vi "Read Channel suffix.vi"(8 "error in (no error)":errorcluster, 11 "Tag Channel Column in":refnum<class "Tag Channel Column.lvclass">) -> (0 "error out":errorcluster, 2 "Channel suffix":string, 3 "Tag Channel Column out":refnum<class "Tag Channel Column.lvclass">)   [LabVIEW 2013, in "Table Manager.lvlib" / "Tag Channel Column.lvclass"]
uses:
  Tag Channel Column.lvclass
  Tag Channel Column.lvclass/Tag Channel Column.ctl
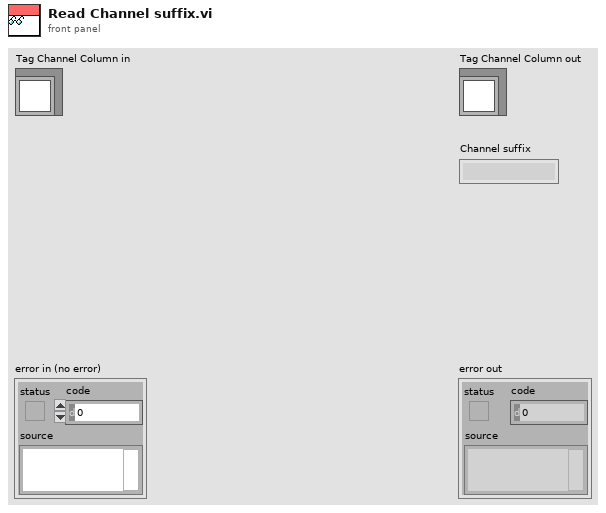
[diagram p1: front panel]
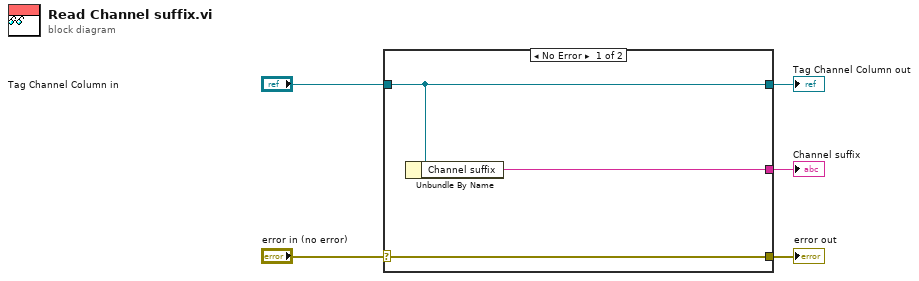
[diagram p0: block diagram]
diagram:
  n1 = case shown="No Error" "error in (no error)" {
    selector: "error in (no error)" -> [w8 w9]
    tunnel: [w8 w9] -> w4
    tunnel: [w7 w10] -> w2
    tunnel: "Tag Channel Column in" -> [w7 w10]
    tunnel: [w6 _] -> w1
    frame No Error {
      n2 = Unbundle By Name(w7) -> ("Channel suffix"=w6:string)
    }
    frame Error {
    }
  }
  "error out" <- w4
  "Tag Channel Column out" <- w2
  "Channel suffix" <- w1
